vi "读取内置参数.vi"(8 "error in (no error)":errorcluster, 11 "MB session in":refnum<class "MB_Master.lvclass">) -> (0 "error out":errorcluster, 1 "float":T1 {"偏心轮校准参数" format="%#.6g"}, 2 "外设配置":T3 {"是否存在液位检测板" items=["否", "是"]; "阀数量" items=["9通"=9, "12通"=12]; "泵类型" items=["TECAN", "润泽"]}, 3 "MB session out":refnum<class "MB_Master.lvclass">, 5 "量程参数读取":T2 {"阈值（高->低）" format="%#.6g"; "阈值（低->高）" format="%#.6g"; "下限" format="%#.6g"; "上限" format="%#.6g"})   [LabVIEW 2016, in "斯坦道CODMn新电路板.lvlib"]
uses:
  <vilib>/Plasmionique/MB Master/MB_Master/MB_Master.lvclass
  <vilib>/Plasmionique/MB Master/MB_Master_Serial/MB_Master_Serial.lvclass
  D:/Program Files (x86)/National Instruments/LabVIEW 2016/vi.lib/Plasmionique/MB Master/MB_Master/MB_Master.lvclass
  <vilib>/Plasmionique/MB Master/MB Master.lvlib
panel:
  in  "VISA Resource":refnum<visa-resource-name>
  in  "引用选择":enum16{"MB引用", "自建引用"}(ring)
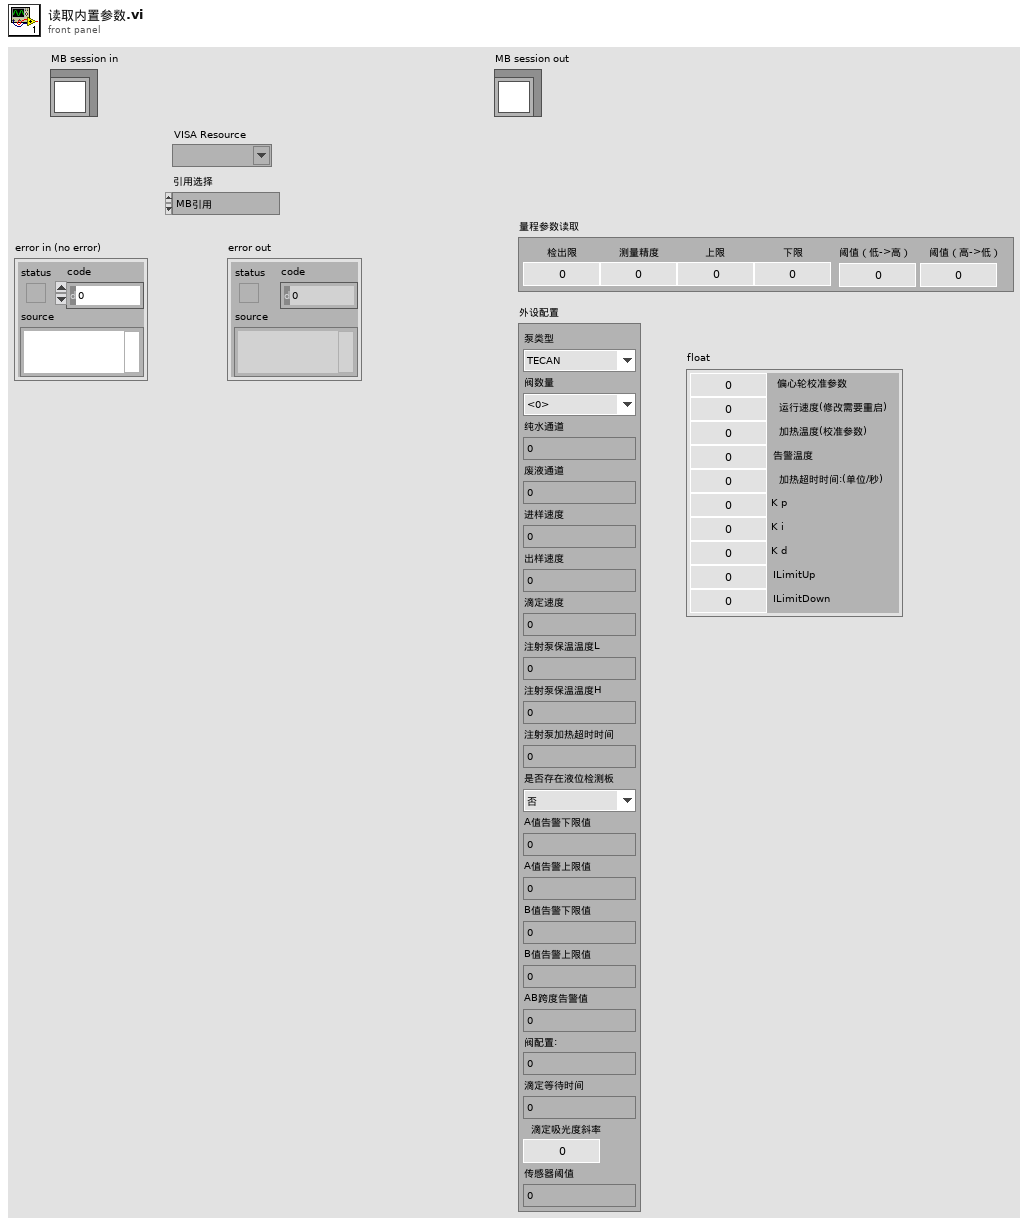
[diagram p1: front panel]
types:
  T1 = cluster{"偏心轮校准参数":dbl, "运行速度(修改需要重启)":u16, "加热温度(校准参数) ":dbl, "告警温度":dbl, "加热超时时间:(单位/秒)":dbl, "K p":dbl, "K i":dbl, "K d":dbl, "ILimitUp":dbl, "ILimitDown":dbl}
  T2 = cluster{"检出限":dbl, "测量精度":dbl, "上限":dbl, "下限":dbl, "阈值（低->高）":dbl, "阈值（高->低）":dbl}
  T3 = cluster{"泵类型":u8, "阀数量":u8, "纯水通道":u16, "废液通道":u8, "进样速度":u16, "出样速度":u16, "滴定速度":u16, "注射泵保温温度L":u8, "注射泵保温温度H":u8, "注射泵加热超时时间":u16, "是否存在液位检测板":u16, "A值告警下限值":u16, "A值告警上限值":u16, "B值告警下限值":u16, "B值告警上限值":u16, "AB跨度告警值":u16, "阀配置:":u8, "滴定等待时间":u16, "滴定吸光度斜率":dbl, "传感器阈值":u16}
  T4 = cluster{"baud rate (bps)":u32, "stop bits":u16, "parity":u16, "flow control":u16, "timeout":u32, "retries":i32}
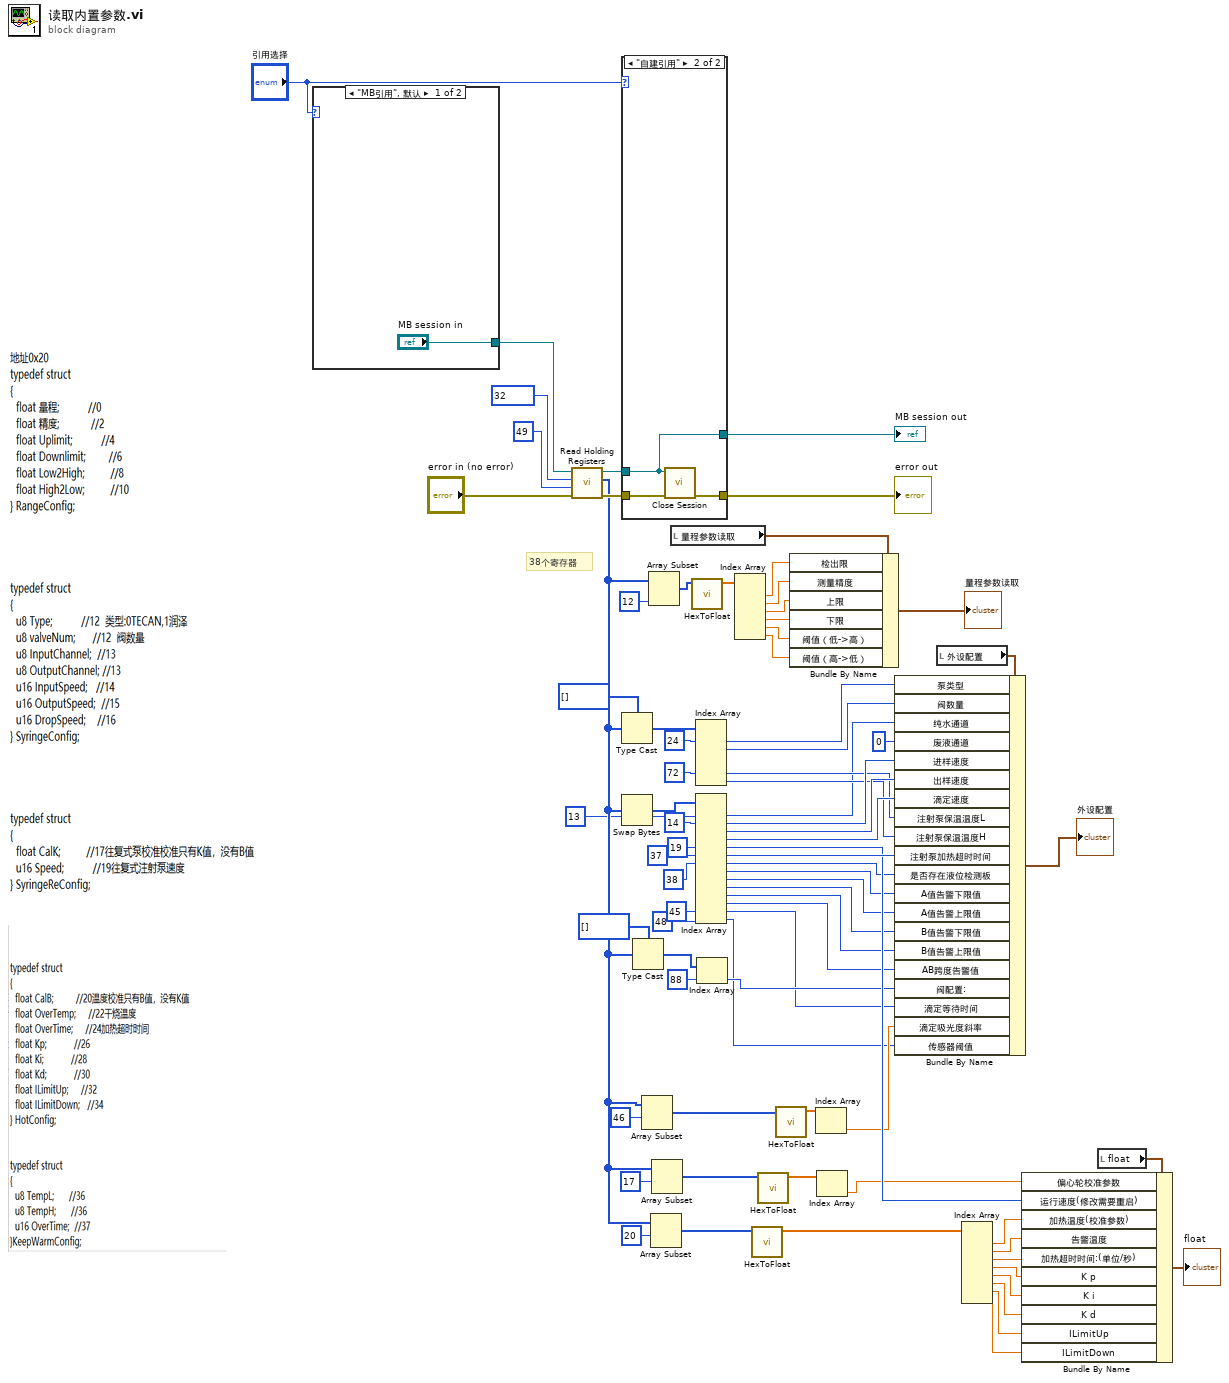
[diagram p0: block diagram]
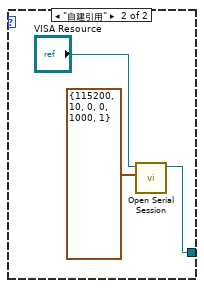
[diagram p3: hidden frame]
diagram:
  # "38个寄存器"
  n1 = case shown="\"MB引用\", 默认" "引用选择" {
    tunnel: ["MB session in" w83] -> w71
    frame "MB引用", Default {
    }
    frame "自建引用" {
      n2 = call <vilib>:"Open Serial Session.vi"("Serial Config"=T4 {"baud rate (bps)"=115200, "stop bits"=10, "parity"=0, "flow control"=0, "timeout"=1000, "retries"=1}, "VISA Resource"="VISA Resource") -> ("MB_Serial session"=w83:refnum<class "MB_Master_Serial.lvclass">)  [unwired: 8 in, 1 out]
    }
  }
  n3 = call <vilib>:"Read Holding Registers.vi"("error in (no error)"="error in (no error)", "quantity"=u16 49, "starting address"=u16 32, "MB session in"=w71) -> ("error out"=w68:errorcluster, "Registers"=w7:u16[], "MB session out"=w70:refnum<class "MB_Master.lvclass">)  [unwired: 5 in]
  n4 = case shown="\"自建引用\"" "引用选择" {
    tunnel: w70 -> [w84 w86]
    tunnel: w68 -> [w85 w88]
    tunnel: [w85 w87] -> w67
    tunnel: [w84 w86] -> w66
    frame "MB引用", Default {
    }
    frame "自建引用" {
      n5 = call-dynamic "Close Session.vi"("error in (no error)"=w88, "MB session in"=w86) -> ("error out"=w87:errorcluster)  [unwired: 9 in]
    }
  }
  "MB session out" <- w66
  "error out" <- w67
  n6 = Type Cast(type=u8[] [], x=w7) -> (*(type *) &x=w72:u8[])
  n7 = Swap Bytes(anything=w7) -> (byte swapped=w47:u16[])
  n8 = Type Cast(type=u8[] [], x=w7) -> (*(type *) &x=w10:u8[])
  n9 = Array Subset(array=w7, index=46 ("索引")) -> (w6:u16[])  [unwired: 1 in]
  n10 = Array Subset(array=w7, length=12 ("长度")) -> (w29:u16[])  [unwired: 1 in]
  n11 = Array Subset(array=w7, index=20 ("索引")) -> (w27:u16[])  [unwired: 1 in]
  n12 = Array Subset(array=w7, index=17 ("索引")) -> (w40:u16[])  [unwired: 1 in]
  n13 = local read "量程参数读取"() -> (w64:T2)
  n14 = call "HexToFloat.vi"("数组"=w29) -> ("FLOAT"=w65:sgl[])  [unwired: 10 in]
  n15 = Index Array(array=w72, index #1=24 ("索引"), index #5=72 ("索引")) -> (element #1=w73:u8, element #2=w56:u8, element #5=w51:u8, element #6=w50:u8)  [unwired: 4 in, 2 out]
  n16 = Index Array(array=w47, index #1=13 ("索引"), index #2=14 ("索引"), index #5=19 ("索引"), index #6=37 ("索引"), index #7=38 ("索引"), index #13=45 ("索引"), index #14=48 ("索引")) -> (element #1=w4:u16, element #2=w55:u16, element #3=w54:u16, element #4=w53:u16, element #5=w39:u16, element #6=w44:u16, element #7=w23:u16, element #8=w21:u16, element #9=w20:u16, element #10=w19:u16, element #11=w18:u16, element #12=w17:u16, element #13=w8:u16, element #14=w1:u16)  [unwired: 7 in]
  n17 = Index Array(array=w10, index=88 ("索引")) -> (element=w14:u8)
  n18 = Index Array(array=w65) -> (element #1=w62:sgl, element #2=w61:sgl, element #3=w60:sgl, element #4=w59:sgl, element #5=w58:sgl, element #6=w57:sgl)  [unwired: 6 in]
  n19 = call "HexToFloat.vi"("数组"=w27) -> ("FLOAT"=w26:sgl[])  [unwired: 10 in]
  n20 = call "HexToFloat.vi"("数组"=w40) -> ("FLOAT"=w25:sgl[])  [unwired: 10 in]
  n21 = call "HexToFloat.vi"("数组"=w6) -> ("FLOAT"=w13:sgl[])  [unwired: 10 in]
  n22 = Bundle By Name(cluster=w64, "检出限"=w62, "测量精度"=w61, "上限"=w60, "下限"=w59, "阈值（低->高）"=w58, "阈值（高->低）"=w57) -> (→"量程参数读取":T2)
  n23 = Index Array(array=w13) -> (element=w11:sgl)  [unwired: 1 in]
  n24 = Index Array(array=w25) -> (element=w24:sgl)  [unwired: 1 in]
  n25 = local read "外设配置"() -> (w75:T3)
  n26 = Bundle By Name(cluster=w75, "泵类型"=w73, "阀数量"=w56, "纯水通道"=w4, "废液通道"=u8 0, "进样速度"=w55, "出样速度"=w54, "滴定速度"=w53, "注射泵保温温度L"=w51, "注射泵保温温度H"=w50, "注射泵加热超时时间"=w44, "是否存在液位检测板"=w23, "A值告警下限值"=w21, "A值告警上限值"=w20, "B值告警下限值"=w19, "B值告警上限值"=w18, "AB跨度告警值"=w17, "阀配置:"=w14, "滴定等待时间"=w8, "滴定吸光度斜率"=w11, "传感器阈值"=w1) -> (→"外设配置":T3)
  n27 = Index Array(array=w26) -> (element #1=w38:sgl, element #2=w37:sgl, element #3=w36:sgl, element #4=w35:sgl, element #5=w34:sgl, element #6=w33:sgl, element #7=w32:sgl, element #8=w31:sgl)  [unwired: 8 in]
  n28 = local read "float"() -> (w43:T1)
  n29 = Bundle By Name(cluster=w43, "偏心轮校准参数"=w24, "运行速度(修改需要重启)"=w39, "加热温度(校准参数)"=w38, "告警温度"=w37, "加热超时时间:(单位/秒)"=w36, "K p"=w35, "K i"=w34, "K d"=w33, "ILimitUp"=w32, "ILimitDown"=w31) -> (→"float":T1)
